vi "Fetch(Y)Trace.vi"(8 "error in (no error)":errorcluster, 11 "SpecAnBase in":refnum<class "SpecAnBase.lvclass">) -> (0 "error out":errorcluster, 3 "SpecAnBase out":refnum<class "SpecAnBase.lvclass">)   [LabVIEW 2014, in "SpecAnPlugins.lvlib" / "SpecAnBase.lvclass"]
doc: "This function returns the trace the spectrum analyzer acquires. The trace is from a previously initiated acquisition. The user calls the Initiate function to start an acquisition. The user calls the Acquisition Status function to determine when the acquisition is complete. \n\nThe user may call the Read Y Trace function instead of the Initiate function. This function starts an acquisition, waits for the acquisition to complete, and returns the trace in one function call. \n\nThe Amplitude array returns data that represents the amplitude of the signals obtained by sweeping from the start frequency to the stop frequency (in frequency domain, in the time domain the amplitude array is ordered from beginning of sweep to end). The Amplitude Units attribute determines the units of the points in the Amplitude array.\n\nThis function does not check the instrument status. The user calls the Error Query function at the conclusion of the sequence to check the instrument status."
uses:
  SpecAnBase.lvclass
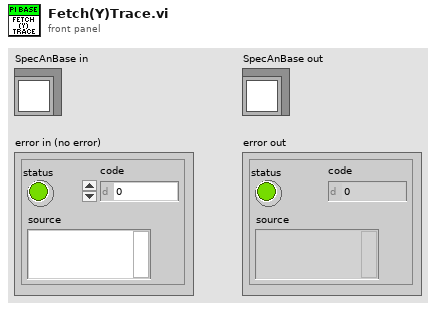
[diagram p1: front panel]
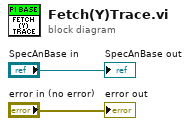
[diagram p0: block diagram]
diagram:
  "error out" <- "error in (no error)"
  "SpecAnBase out" <- "SpecAnBase in"
